vi "Configure Resistance Leakage Guard.vi"(8 "error in (no error)":errorcluster, 10 "Enable Resistance Guard (F: Disable)":bool, 11 "VISA resource name":refnum<visa-resource-name>) -> (0 "error out":errorcluster, 3 "VISA resource name out":refnum<visa-resource-name>)   [LabVIEW 2019, in "Keithley 6517.lvlib"]
doc: "Enables or Disables Resistance leakage (driven) guard.\n\nThe purpose of guarding is to eliminate the effects of leakage resistance and capacitance, that can exist between input HI and input LO. This leakage resistance and capacitance could\nadversely affect high-impedance measurements.\n\n<B>Note:</B>\nThis VI is ONLY compatible with <B>model 6514</B>. Running this Vi with any other model will result in an error."
uses:
  Keithley 6517.lvlib
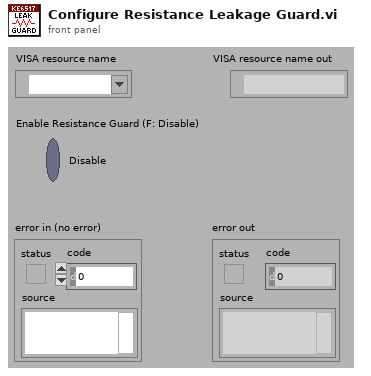
[diagram p1: front panel]
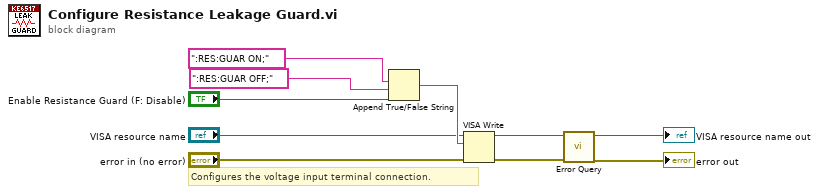
[diagram p0: block diagram]
diagram:
  # "Configures the voltage input terminal connection."
  n1 = Append True/False String(1:"Enable Resistance Guard (F: Disable)", 2:":RES:GUAR OFF;", 3:":RES:GUAR ON;") -> (0:w7:string)  [unwired: 1 in]
  n2 = VISA Write(VISA resource name="VISA resource name", write buffer=w7, error in (no error)="error in (no error)") -> (VISA resource name out=w4:refnum<visa-resource-name>, error out=w3:errorcluster)  [unwired: 1 out]
  n3 = call "Error Query.vi"("error in (no error)"=w3, "VISA resource name"=w4) -> ("error out"=→"error out":errorcluster, "VISA resource name out"=→"VISA resource name out":refnum<visa-resource-name>)  [unwired: 6 in, 2 out]
